vi "3458A Fetch from Digitizing Process.vi"(6 "stop ref":refnum<vi>, 7 "record start timestamp for time multiplex [s]":dbl, 8 "error in":errorcluster, 10 "Is last multiplexing cycle? (True)":bool=TRUE, 11 "session in":T3={"channels"=[], "sync unit"={"VISA"="", "type"=enum."Picotest U6200A"}, "awg unit"={"type"=enum."Agilent 331xxA to 332xxA", "VISA"="", "enable 10MHz ref"=FALSE, "cmi ckd2"={"VISA"="", "clock source"=enum."Auto", "manual ref clk"=FALSE, "ref clock [Hz]"=0.0, "div mode"=enum."Set divisor directly"}, "cmi sync v3"={"VISA"="", "baud rate [bd/s]"=115200, "source"=enum."Auto", "hv range"=enum."1kV", "fsrc is fixed"=FALSE, "fsrc [Hz]"=10000000.0, "freq integ [s]"=1.0, "freq filter"=5, "trig level"=enum."TTL 5V", "chn1 mode"=enum."Source divider", "chn1 level"=enum."Positive 5V", "chn2 mode"=enum."Source divider", "chn2 level"=enum."Positive 5V", "chn2 div"=1, "chn3 mode"=enum."Chn 1 Active", "chn3 level"=enum."Positive 5V", "chn1 div entry"=enum."Calculate nearest divisor from measured fx", "chn1 dev limit [%]"=1.0, "chn1 check dev"=FALSE}, "trigger"={"source"=enum."Immediate", "slope"=enum."POS", "coupling"=enum."DC", "level [V]"=0.0, "hysteresis [V]"=0.0, "pre-trigger [%]"=0.0}, "HMF2500 cfg"={"Baud Rate"=9600, "Parity"=0, "Data Bits"=8, "Flow Control"=4}}, "sync mode"=enum."MASTER-SLAVE, MASTER clocked by TIMER", "streaming mode"=FALSE, "idn mode"=enum."Auto", "sampling mode"=enum."DCV", "sample memory [B]"=0, "proc setup"={"channel id"=0, "packet size [smpl]"=0, "current timeout [s]"=0.0, "blk2blk timeout [s]"=0.0, "event time"=timestamp(0 s since 1904-01-01), "stop notifier"=refnum, "data queues"=[], "proc refs"=[], "bus semaphore"=refnum}, "sample size [B]"=0, "sample count"=0, "aux data"={"channel id"=0, "valid?"=[], "gain [V]"=[], "timestamp [s]"=[], "Ts [s]"=0.0, "abs timestamp"=timestamp(0 s since 1904-01-01), "t [deg C]"=[], "multiplex timestamp [s]"=-1.0, "only multiplex?"=FALSE, "multiplex smpl offset"=0, "overflow?"=FALSE}, "ranges [V]"=[], "aperture [s]"=0.0, "LEVEL trigger"={"edge"=enum."POS", "level [V]"=0.0, "coupling"=enum."DC"}, "trigger mode"=enum."AUTO", "measure temp.?"=FALSE, "disp mesages"=[], "shared bus?"=FALSE, "disable display?"=FALSE, "aper mode"=enum."Manual", "aper rules"=[], "multiplex"={"cycles"=0, "delay [s]"=0.0, "enabled"=FALSE, "overhead [s]"=1.0, "tot smpls"=0, "sub-rec"=0, "overhead [%]"=0.0, "emulated"=FALSE}, "F8588 lpf"=enum."Off", "F8588 pll"=enum."Off", "F8588 couple"=enum."DC, auto", "fs"={"freq mode"=enum."fs or Ts", "fs [Hz]"=0.0, "fref [Hz]"=0.0, "mul"=0.0, "div"=0.0}, "fs mode"=enum."fs or Ts"} {"awg unit"."HMF2500 cfg"."Flow Control" items=["None", "XON/XOFF", "RTS/CTS", "XON/XOFF & RTS/CTS", "DTR/DSR", "XON/XOFF & DTR/DSR"]; "awg unit"."HMF2500 cfg"."Data Bits" items=["7"=7, "8"=8]; "awg unit"."HMF2500 cfg"."Parity" items=["None", "Odd", "Even", "Mark", "Space"]; "awg unit"."HMF2500 cfg"."Baud Rate" items=["300"=300, "600"=600, "1200"=1200, "2400"=2400, "4800"=4800, "9600"=9600, "19200"=19200]; "awg unit"."cmi sync v3"."chn2 div" min=1 max=100000000 step=1; "awg unit"."cmi sync v3"."fsrc [Hz]" format="%_8p"; "channels"."Range [Vpk]" min=0.0}) -> (0 "error out":errorcluster, 1 "aux data":T1={"channel id"=0, "valid?"=[], "gain [V]"=[], "timestamp [s]"=[], "Ts [s]"=0.0, "abs timestamp"=timestamp(0 s since 1904-01-01), "t [deg C]"=[], "multiplex timestamp [s]"=-1.0, "only multiplex?"=FALSE, "multiplex smpl offset"=0, "overflow?"=FALSE}, 2 "data packet":T2, 3 "session out":T3={"channels"=[], "sync unit"={"VISA"="", "type"=enum."Picotest U6200A"}, "awg unit"={"type"=enum."Agilent 331xxA to 332xxA", "VISA"="", "enable 10MHz ref"=FALSE, "cmi ckd2"={"VISA"="", "clock source"=enum."Auto", "manual ref clk"=FALSE, "ref clock [Hz]"=0.0, "div mode"=enum."Set divisor directly"}, "cmi sync v3"={"VISA"="", "baud rate [bd/s]"=115200, "source"=enum."Auto", "hv range"=enum."1kV", "fsrc is fixed"=FALSE, "fsrc [Hz]"=10000000.0, "freq integ [s]"=1.0, "freq filter"=5, "trig level"=enum."TTL 5V", "chn1 mode"=enum."Source divider", "chn1 level"=enum."Positive 5V", "chn2 mode"=enum."Source divider", "chn2 level"=enum."Positive 5V", "chn2 div"=1, "chn3 mode"=enum."Chn 1 Active", "chn3 level"=enum."Positive 5V", "chn1 div entry"=enum."Calculate nearest divisor from measured fx", "chn1 dev limit [%]"=1.0, "chn1 check dev"=FALSE}, "trigger"={"source"=enum."Immediate", "slope"=enum."POS", "coupling"=enum."DC", "level [V]"=0.0, "hysteresis [V]"=0.0, "pre-trigger [%]"=0.0}, "HMF2500 cfg"={"Baud Rate"=9600, "Parity"=0, "Data Bits"=8, "Flow Control"=4}}, "sync mode"=enum."MASTER-SLAVE, MASTER clocked by TIMER", "streaming mode"=FALSE, "idn mode"=enum."Auto", "sampling mode"=enum."DCV", "sample memory [B]"=0, "proc setup"={"channel id"=0, "packet size [smpl]"=0, "current timeout [s]"=0.0, "blk2blk timeout [s]"=0.0, "event time"=timestamp(0 s since 1904-01-01), "stop notifier"=refnum, "data queues"=[], "proc refs"=[], "bus semaphore"=refnum}, "sample size [B]"=0, "sample count"=0, "aux data"={"channel id"=0, "valid?"=[], "gain [V]"=[], "timestamp [s]"=[], "Ts [s]"=0.0, "abs timestamp"=timestamp(0 s since 1904-01-01), "t [deg C]"=[], "multiplex timestamp [s]"=-1.0, "only multiplex?"=FALSE, "multiplex smpl offset"=0, "overflow?"=FALSE}, "ranges [V]"=[], "aperture [s]"=0.0, "LEVEL trigger"={"edge"=enum."POS", "level [V]"=0.0, "coupling"=enum."DC"}, "trigger mode"=enum."AUTO", "measure temp.?"=FALSE, "disp mesages"=[], "shared bus?"=FALSE, "disable display?"=FALSE, "aper mode"=enum."Manual", "aper rules"=[], "multiplex"={"cycles"=0, "delay [s]"=0.0, "enabled"=FALSE, "overhead [s]"=1.0, "tot smpls"=0, "sub-rec"=0, "overhead [%]"=0.0, "emulated"=FALSE}, "F8588 lpf"=enum."Off", "F8588 pll"=enum."Off", "F8588 couple"=enum."DC, auto", "fs"={"freq mode"=enum."fs or Ts", "fs [Hz]"=0.0, "fref [Hz]"=0.0, "mul"=0.0, "div"=0.0}, "fs mode"=enum."fs or Ts"} {"awg unit"."HMF2500 cfg"."Flow Control" items=["None", "XON/XOFF", "RTS/CTS", "XON/XOFF & RTS/CTS", "DTR/DSR", "XON/XOFF & DTR/DSR"]; "awg unit"."HMF2500 cfg"."Data Bits" items=["7"=7, "8"=8]; "awg unit"."HMF2500 cfg"."Parity" items=["None", "Odd", "Even", "Mark", "Space"]; "awg unit"."HMF2500 cfg"."Baud Rate" items=["300"=300, "600"=600, "1200"=1200, "2400"=2400, "4800"=4800, "9600"=9600, "19200"=19200]; "awg unit"."cmi sync v3"."chn2 div" min=1 max=100000000 step=1; "awg unit"."cmi sync v3"."fsrc [Hz]" format="%_8p"; "channels"."Range [Vpk]" min=0.0}, 4 "fetching done?":bool)   [LabVIEW 2020, in "3458A Virtual Digitizer.lvlib"]
doc: "This VI fetches digitized samples from the digitizing processes initiated by 'Initiate Digitizing Process'. It checks the data queues of the particular channels and merges samples from the channels into 2D array whenever all channels return matching series of samples. Until all channels sends some samples to the queues it won't return data but also won't return error. When some of the digitizing processes exits with error or exits prematurely it will generate error. It will also generate error when fetching timeout occures. When processes seems to returnes unsynchronized data it will also generate error and terminate fetching. Called of this vi must keep checking flag 'valid?' in the 'data packet' and 'aux data'. When the flag is True the data must be checked/collected. When this VI returnes 'fetching done?' or error flag the caller shall not call the function again.\n\nFor multiplexing mode and not 'Is last multiplex cycle?' it will only wait to emulate recording and returns 'Fetching done'. It will only fetch in the last multiplex cycle (default)."
uses:
  3458A Virtual Digitizer.lvlib
  3458A Digitizer Session.ctl
  3458A Virtual Channel Config.ctl
  Counter/Counter Session.ctl
  Counter/Counter Type.ctl
  AWG/AWG Session.ctl
  AWG/AWG Type.ctl
  AWG/CMI Clock Divider v2/CMI ckd2 Session.ctl
  AWG/CMI Clock Divider v2/CMI ckd2 Source Mode.ctl
  AWG/CMI Clock Divider v2/CMI ckd2 Divisor Mode.ctl
  AWG/CMI Sync V3/CMI Sync V3 session.ctl
  AWG/CMI Sync V3/Configure/CMI Sync V3 Reference Clock Source.ctl
  AWG/CMI Sync V3/Configure/CMI Sync V3 HV input Range.ctl
  AWG/CMI Sync V3/Configure/CMI Sync V3 Trigger Input Level.ctl
  AWG/CMI Sync V3/Configure/CMI Sync V3 Channel 1 Mode.ctl
  AWG/CMI Sync V3/Configure/CMI Sync V3 Channel Output Levels.ctl
  AWG/CMI Sync V3/Configure/CMI Sync V3 Channel 2 Mode.ctl
  AWG/CMI Sync V3/Configure/CMI Sync V3 Channel 3 Mode.ctl
  AWG/CMI Sync V3/Configure/CMI Sync V3 Channel 1 Divisor Entry Mode.ctl
  adc/ADC Trig Config.ctl
  adc/ADC Trig Mode Source.ctl
  adc/ADC Trig Slope.ctl
  adc/ADC Trig Coupling.ctl
  AWG/RaS HMF2500/HMF2500 Config.ctl
  3458A Sync Mode.ctl
  3458A Idn Mode.ctl
  3458A Digitizing Low Levels/Configure/Sampling Mode.ctl
  3458A Digitizing Process Options.ctl
  3458A Data Packet.ctl
  3458A Aux Record Data.ctl
  3458A Digitizing Low Levels/Configure/Level Setup.ctl
  3458A Digitizing Low Levels/Configure/First Sample Trigger.ctl
  3458A Aperture Selection Mode.ctl
  3458A Multiplexing Config.ctl
  Fluke 8588A/F8588A Low Pass Filter.ctl
  Fluke 8588A/F8588A Phase Lock.ctl
  Fluke 8588A/F8588A Coupling.ctl
  3458A Sampling Rate.ctl
  AWG/AWG Clock Setup Mode.ctl
  3458A Sample Rate Mode.ctl
  <vilib>/Utility/error.llb/Error Cluster From Error Code.vi
  <vilib>/ErrorRing/Error Ring.xnode
  varilib/varilib.lvlib
  AWG/AWG.lvlib
  Counter/Counter.lvlib
  3458A Digitizing Low Levels/3458A Digitizing Low Levels.lvlib
  AWG/CMI Sync V3/CMI Sync Unit V3.lvlib
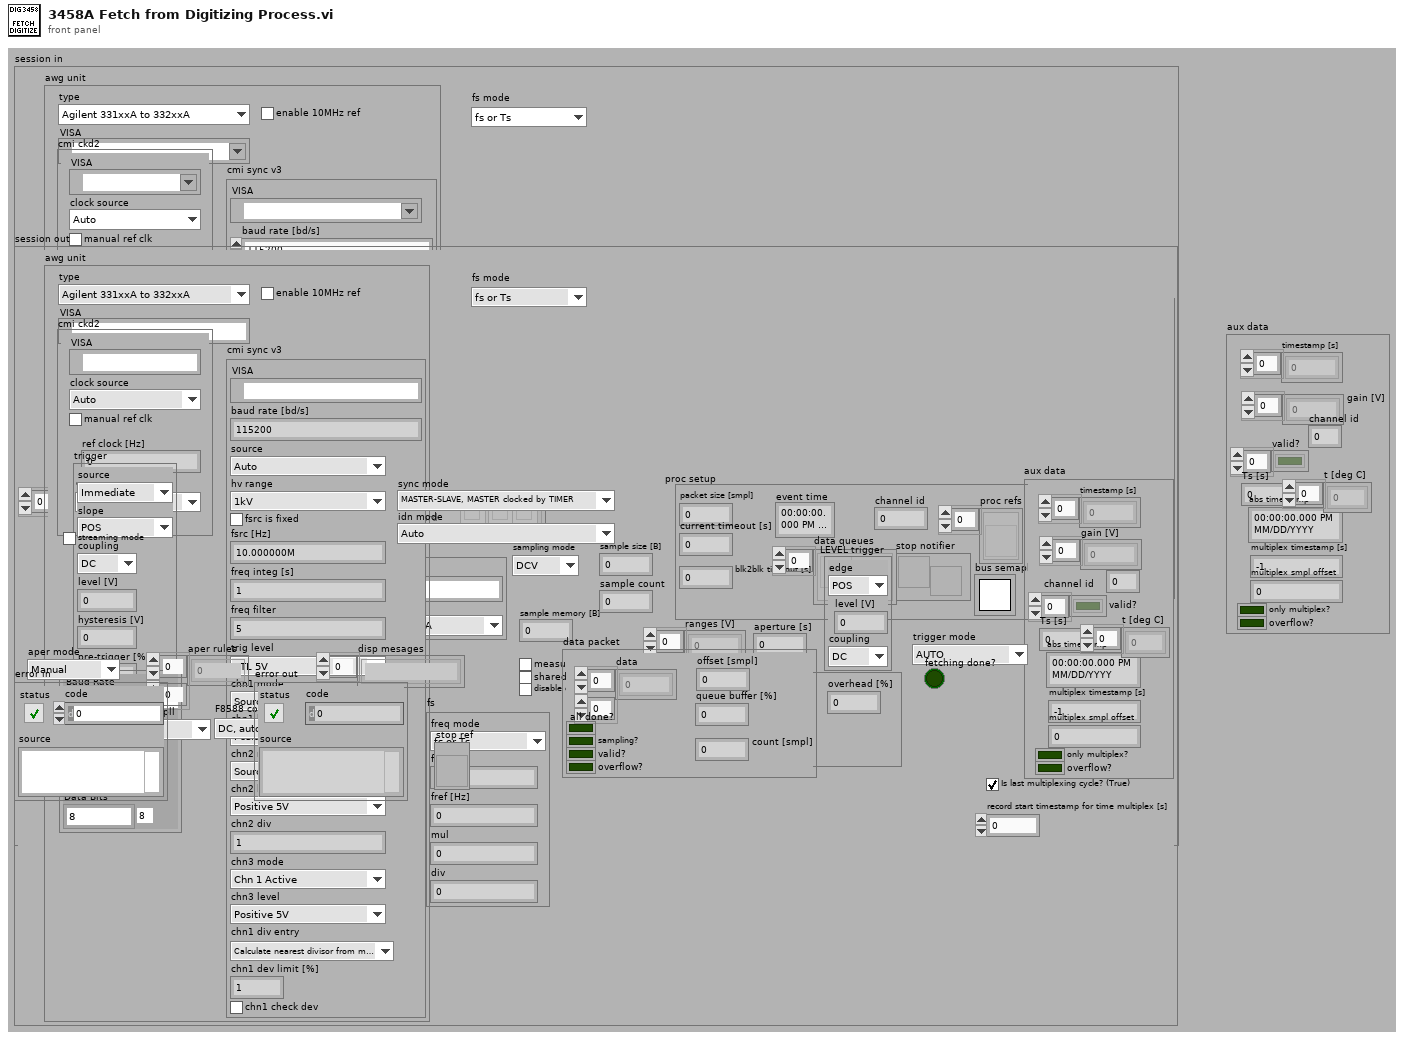
[diagram p1: front panel]
types:
  T1 = typedef "3458A Virtual Digitizer.lvlib/3458A Aux Record Data.ctl" = cluster{"channel id":i32, "valid?":bool[], "gain [V]":dbl[], "timestamp [s]":dbl[], "Ts [s]":dbl, "abs timestamp":timestamp, "t [deg C]":dbl[], "multiplex timestamp [s]":dbl, "only multiplex?":bool, "multiplex smpl offset":i64, "overflow?":bool}
  T2 = typedef "3458A Virtual Digitizer.lvlib/3458A Data Packet.ctl" = cluster{"data":i32[][], "offset [smpl]":i32, "count [smpl]":i32, "all done?":bool, "sampling?":bool, "queue buffer [%]":dbl, "valid?":bool, "overflow?":bool}
  T3 = typedef "3458A Virtual Digitizer.lvlib/3458A Digitizer Session.ctl" = cluster{"channels":T4[], "sync unit":T5, "awg unit":T7, "sync mode":T26, "streaming mode":bool, "idn mode":T27, "sampling mode":T28, "sample memory [B]":i32, "proc setup":T29, "sample size [B]":i32, "sample count":i32, "aux data":T1, "ranges [V]":dbl[], "aperture [s]":dbl, "LEVEL trigger":T31, "trigger mode":T32, "measure temp.?":bool, "disp mesages":string[], "shared bus?":bool, "disable display?":bool, "aper mode":T33, "aper rules":dbl[][], "multiplex":T34, "F8588 lpf":T35, "F8588 pll":T36, "F8588 couple":T37, "fs":T38, "fs mode":T40}
  T4 = typedef "3458A Virtual Digitizer.lvlib/3458A Virtual Channel Config.ctl" = cluster{"VISA":refnum<visa-resource-name>, "Range [Vpk]":dbl, "btn clr":bool, "btn up":bool, "btn down":bool, "F8588":bool, "F8588 guard":bool}
  T5 = typedef "Counter.lvlib/Counter Session.ctl" = cluster{"VISA":refnum<visa-resource-name>, "type":T6}
  T6 = typedef "Counter.lvlib/Counter Type.ctl" = enum16{"Picotest U6200A", "dummy"}
  T7 = typedef "AWG.lvlib/AWG Session.ctl" = cluster{"type":T8, "VISA":refnum<visa-resource-name>, "enable 10MHz ref":bool, "cmi ckd2":T9, "cmi sync v3":T12, "trigger":T21, "HMF2500 cfg":T25}
  T8 = typedef "AWG.lvlib/AWG Type.ctl" = enum16{"Agilent 331xxA to 332xxA", "Agilent 335xxA to 336xxA", "Tektronix AFG3101C", "R&S HMF25xx", "CMI Clock Divider v2", "CMI Sync Unit V3", "dummy"}
  T9 = typedef "AWG.lvlib/CMI ckd2 Session.ctl" = cluster{"VISA":refnum<visa-resource-name>, "clock source":T10, "manual ref clk":bool, "ref clock [Hz]":dbl, "div mode":T11}
  T10 = typedef "AWG.lvlib/CMI ckd2 Source Mode.ctl" = enum16{"Auto", "LF clock", "HF clock", "Internal"}
  T11 = typedef "AWG.lvlib/CMI ckd2 Divisor Mode.ctl" = enum16{"Set divisor directly", "Set divisor by frequency"}
  T12 = typedef "AWG.lvlib/CMI Sync Unit V3.lvlib/CMI Sync V3 session.ctl" = cluster{"VISA":refnum<visa-resource-name>, "baud rate [bd/s]":i32, "source":T13, "hv range":T14, "fsrc is fixed":bool, "fsrc [Hz]":dbl, "freq integ [s]":dbl, "freq filter":i32, "trig level":T15, "chn1 mode":T16, "chn1 level":T17, "chn2 mode":T18, "chn2 level":T17, "chn2 div":i32, "chn3 mode":T19, "chn3 level":T17, "chn1 div entry":T20, "chn1 dev limit [%]":dbl, "chn1 check dev":bool}
  T13 = typedef "AWG.lvlib/CMI Sync Unit V3.lvlib/CMI Sync V3 Reference Clock Source.ctl" = enum16{"Auto", "Internal", "Logic", "Sine", "HV"}
  T14 = typedef "AWG.lvlib/CMI Sync Unit V3.lvlib/CMI Sync V3 HV input Range.ctl" = enum16{"10V", "60V", "250V", "1kV"}
  T15 = typedef "AWG.lvlib/CMI Sync Unit V3.lvlib/CMI Sync V3 Trigger Input Level.ctl" = enum16{"LVCMOS 3V3", "TTL 5V"}
  T16 = typedef "AWG.lvlib/CMI Sync Unit V3.lvlib/CMI Sync V3 Channel 1 Mode.ctl" = enum16{"Source divider", "DDS absolute", "DDS ratio", "DDS ratio M/N"}
  T17 = typedef "AWG.lvlib/CMI Sync Unit V3.lvlib/CMI Sync V3 Channel Output Levels.ctl" = enum16{"Positive 3V3", "Negative 3V3", "Positive 5V", "Negative 5V"}
  T18 = typedef "AWG.lvlib/CMI Sync Unit V3.lvlib/CMI Sync V3 Channel 2 Mode.ctl" = enum16{"Source divider", "Chn 1 divide"}
  T19 = typedef "AWG.lvlib/CMI Sync Unit V3.lvlib/CMI Sync V3 Channel 3 Mode.ctl" = enum16{"Chn 1 Active", "Chn 2 Active", "Chn 1 Trigger", "Chn 2 Trigger", "Gate", "PPS", "10MHz"}
  T20 = typedef "AWG.lvlib/CMI Sync Unit V3.lvlib/CMI Sync V3 Channel 1 Divisor Entry Mode.ctl" = enum16{"Set divisor directly", "Calculate nearest divisor from measured fx"}
  T21 = typedef "ADC Trig Config.ctl" = cluster{"source":T22, "slope":T23, "coupling":T24, "level [V]":dbl, "hysteresis [V]":dbl, "pre-trigger [%]":dbl}
  T22 = typedef "ADC Trig Mode Source.ctl" = enum16{"Immediate", "External", "Level"}
  T23 = typedef "ADC Trig Slope.ctl" = enum16{"POS", "NEG"}
  T24 = typedef "ADC Trig Coupling.ctl" = enum16{"DC", "AC"}
  T25 = typedef "AWG.lvlib/HMF2500 Config.ctl" = cluster{"Baud Rate":u32, "Parity":u16, "Data Bits":u16, "Flow Control":u16}
  T26 = typedef "3458A Virtual Digitizer.lvlib/3458A Sync Mode.ctl" = enum16{"MASTER-SLAVE, MASTER clocked by TIMER", "MASTER-SLAVE, MASTER clocked by AWG", "ALL clocked by AWG", "MASTER-SLAVE, ALL clocked by TIMER", "ALL clocked by AWG with DFLL"}
  T27 = typedef "3458A Virtual Digitizer.lvlib/3458A Idn Mode.ctl" = enum16{"Auto", "Sequential (chn A, chn B, ...)", "From calibration string"}
  T28 = typedef "3458A Virtual Digitizer.lvlib/3458A Digitizing Low Levels.lvlib/Sampling Mode.ctl" = enum16{"DCV", "DSDC", "DSAC"}
  T29 = typedef "3458A Virtual Digitizer.lvlib/3458A Digitizing Process Options.ctl" = cluster{"channel id":i32, "packet size [smpl]":i32, "current timeout [s]":dbl, "blk2blk timeout [s]":dbl, "event time":timestamp, "stop notifier":refnum<notifier>, "data queues":refnum<queue>[], "proc refs":refnum<vi>[], "bus semaphore":T30}
  T30 = typedef "Semaphore RefNum" = refnum<k1>
  T31 = typedef "3458A Virtual Digitizer.lvlib/3458A Digitizing Low Levels.lvlib/Level Setup.ctl" = cluster{"edge":enum16{"POS", "NEG"}, "level [V]":dbl, "coupling":enum16{"DC", "AC"}}
  T32 = typedef "3458A Virtual Digitizer.lvlib/3458A Digitizing Low Levels.lvlib/First Sample Trigger.ctl" = enum16{"AUTO", "EXT", "SYN", "SGL", "HOLD", "LEVEL"}
  T33 = typedef "3458A Virtual Digitizer.lvlib/3458A Aperture Selection Mode.ctl" = enum16{"Manual", "Maximum", "Table"}
  T34 = typedef "3458A Virtual Digitizer.lvlib/3458A Multiplexing Config.ctl" = cluster{"cycles":i32, "delay [s]":dbl, "enabled":bool, "overhead [s]":dbl, "tot smpls":i64, "sub-rec":i32, "overhead [%]":dbl, "emulated":bool}
  T35 = typedef "F8588A Low Pass Filter.ctl" = enum16{"Off", "100 kHz", "3 MHz"}
  T36 = typedef "F8588A Phase Lock.ctl" = enum16{"Off", "1 MHz", "10 MHz"}
  T37 = typedef "F8588A Coupling.ctl" = enum16{"AC, 1 MOhm", "AC, 10 MOhm", "DC, 1 MOhm", "DC, 10 MOhm", "DC, auto"}
  T38 = typedef "3458A Virtual Digitizer.lvlib/3458A Sampling Rate.ctl" = cluster{"freq mode":T39, "fs [Hz]":dbl, "fref [Hz]":dbl, "mul":dbl, "div":dbl}
  T39 = typedef "AWG.lvlib/AWG Clock Setup Mode.ctl" = enum16{"fs or Ts", "fs or Ts with fref", "fref/N", "fref*M/N", "fref*Ratio"}
  T40 = typedef "3458A Sample Rate Mode.ctl" = enum16{"fs or Ts", "fs*M/N"}
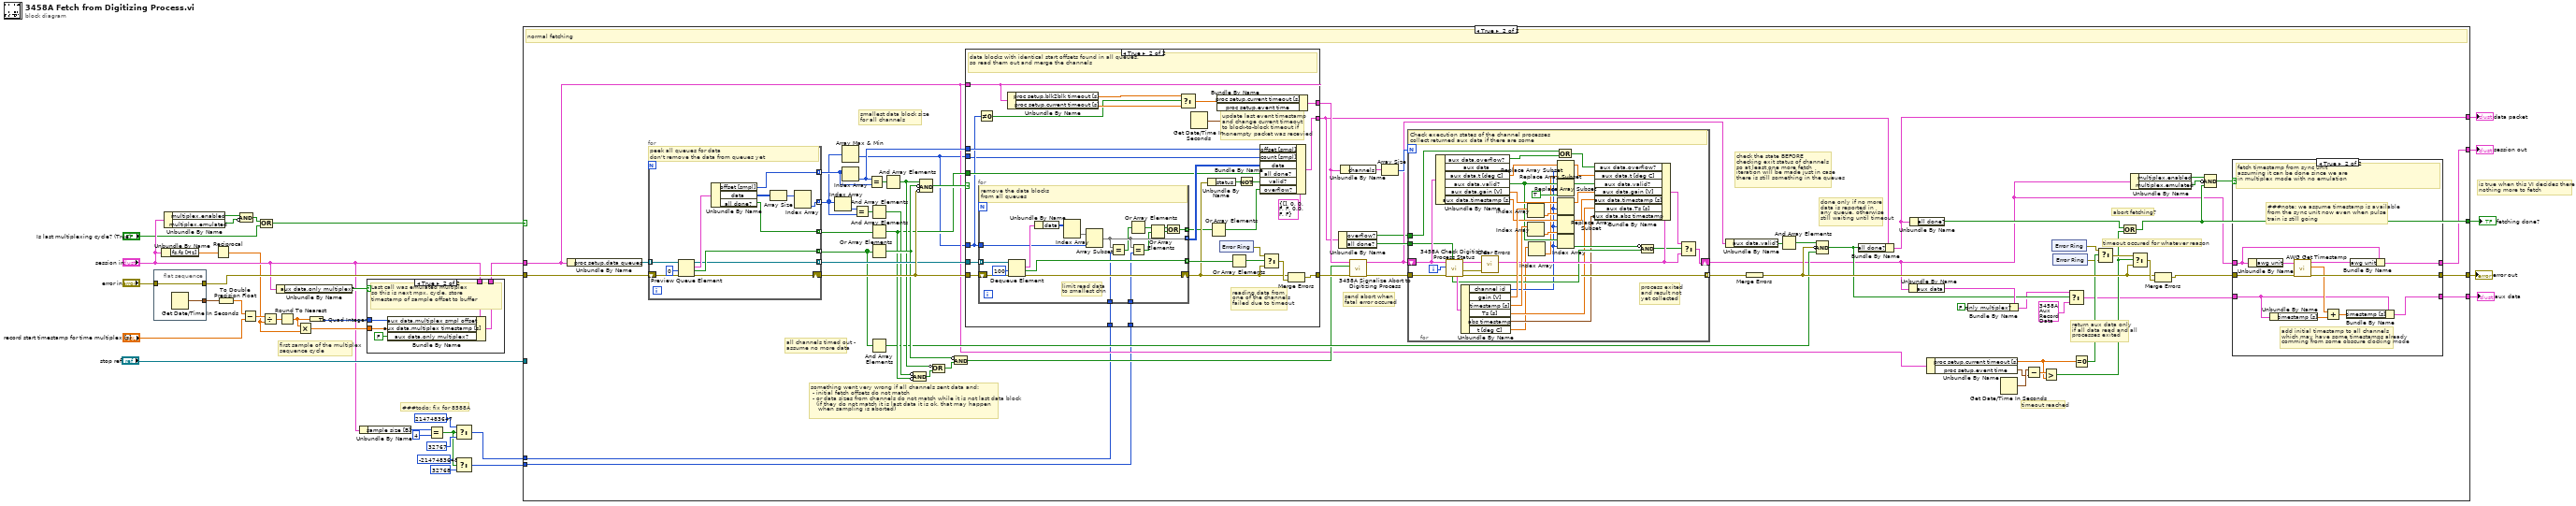
[diagram p0: block diagram]
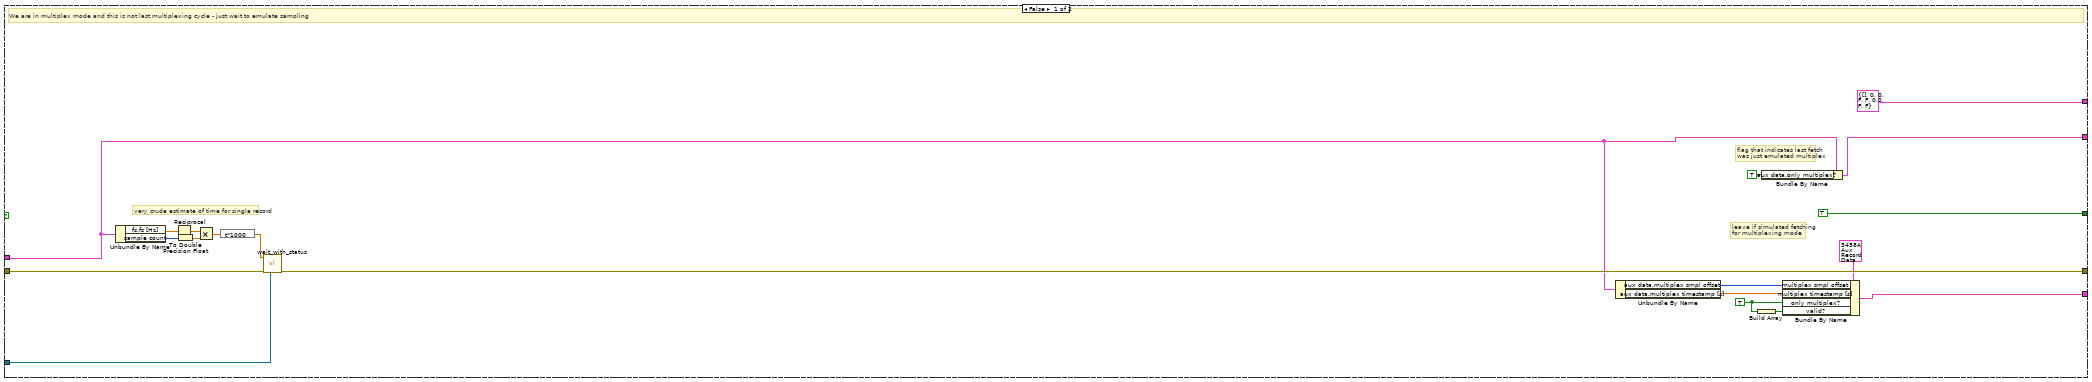
[diagram p3: hidden frame]
diagram:
  # "###todo: fix for 8588A"
  # "first sample of the multiplex\nsequence cycle"
  # "is true when this VI decides there is\nnothing more to fetch"
  n1 = flat-sequence {
    tunnel: [w37] -> w23
    tunnel: "error in" -> [w37]
    tunnel: [w36] -> w26
    frame #0 {
      n2 = Get Date/Time In Seconds() -> (seconds since 1Jan1904=w36:timestamp)
    }
  }
  n3 = Unbundle By Name("session in") -> ("fs.fs [Hz]"=w21:dbl)
  n4 = Unbundle By Name("session in") -> ("multiplex.enabled"=w6:bool, "multiplex.emulated"=w5:bool)
  n5 = Reciprocal(x=w21) -> (1/x=w1:dbl)
  n6 = To Double Precision Float(number=w26) -> (double precision float=w27:dbl)
  n7 = Compound Arithmetic op=AND(w6, invert w5) -> (w4:bool)
  n8 = Subtract(x=w27, y="record start timestamp for time multiplex [s]") -> (x-y=w28:dbl)
  n9 = Compound Arithmetic op=OR(w4, "Is last multiplexing cycle? (True)") -> (w2:bool)
  n10 = Divide(x=w28, y=w1) -> (x/y=w29:dbl)
  n11 = Unbundle By Name("session in") -> ("aux data.only multiplex?"=w19:bool)
  n12 = Round To Nearest(number=w29) -> (nearest integer value=w22:dbl)
  n13 = Multiply(x=w22, y=w1) -> (x*y=w17:dbl)
  n14 = To Quad Integer(1:w22) -> (0:w18:i64)
  n15 = Unbundle By Name("session in") -> ("sample size [B]"=w16:i32)
  n16 = case shown="True" w19 {
    tunnel: "session in" -> [w38 w43]
    tunnel: [w38 w42] -> w20
    tunnel: w18 -> [_ w40]
    tunnel: w17 -> [_ w39]
    frame False {
      # "regular fetch - do nothing"
    }
    frame True {
      # "Last call was emulated multiplex\nso this is next mpx. cycle, store\ntimestamp of sample offset to buffer"
      n17 = Bundle By Name(cluster=w43, "aux data.multiplex smpl offset"=w40, "aux data.multiplex timestamp [s]"=w39, "aux data.only multiplex?"=FALSE) -> (w42:T3)
    }
  }
  n18 = Equal?(x=w16, y=4) -> (x = y?=w12:bool)
  n19 = Select(t=2147483647 ("y"), s=w12, f=32767 ("y")) -> (s? t:f=w8:i32)
  n20 = Select(t=-2147483648 ("y"), s=w12, f=32768 ("y")) -> (s? t:f=w9:i32)
  n21 = case shown="True" w2 {
    tunnel: w23 -> [w56 w128]
    tunnel: [w60 w70] -> w35
    tunnel: w20 -> [w49 w81]
    tunnel: [w51 w66] -> w34
    tunnel: "stop ref" -> [w59 _]
    tunnel: [TRUE w68] -> w32
    tunnel: [w54 w64] -> w31
    tunnel: [T2 {"data"=[], "offset [smpl]"=0, "count [smpl]"=0, "all done?"=FALSE, "sampling?"=FALSE, "queue buffer [%]"=0.0, "valid?"=FALSE, "overflow?"=FALSE} ("niScope packet") w79] -> w30
    tunnel: w9 -> [_ w75]
    tunnel: w8 -> [_ w76]
    frame False {
      w52 = TRUE ("only multiplex?")
      # "flag that indicates last fetch\nwas just emulated multiplex"
      # "leave if simulated fetching\nfor multiplexing mode"
      # "very crude estimate of time for single record"
      # "We are in multiplex mode and this is not last multiplexing cycle - just wait to emulate sampling"
      n22 = Unbundle By Name(w49) -> ("fs.fs [Hz]"=w57:dbl, "sample count"=w63:i32)
      n23 = Reciprocal(x=w57) -> (1/x=w44:dbl)
      n24 = To Double Precision Float(number=w63) -> (double precision float=w62:dbl)
      n25 = Multiply(x=w44, y=w62) -> (x*y=w61:dbl)
      n26 = expression code="t*1000"(w61) -> (w45:dbl)
      n27 = call "wait_with_status.vi"("stop ref"=w59, "error in"=w56, "ms to wait"=w45) -> ("error out"=w60:errorcluster)  [unwired: 8 in]
      n28 = Unbundle By Name(w49) -> ("aux data.multiplex smpl offset"=w48:i64, "aux data.multiplex timestamp [s]"=w47:dbl)
      n29 = Build Array(w52) -> (w53:bool[])
      n30 = Bundle By Name(cluster=w49, "aux data.only multiplex?"=TRUE) -> (w51:T3)
      n31 = Bundle By Name(cluster=T1 {"channel id"=0, "valid?"=[], "gain [V]"=[], "timestamp [s]"=[], "Ts [s]"=0.0, "abs timestamp"=timestamp(0 s since 1904-01-01), "t [deg C]"=[], "multiplex timestamp [s]"=0.0, "only multiplex?"=FALSE, "multiplex smpl offset"=0, "overflow?"=FALSE} ("f"), "multiplex smpl offset"=w48, "multiplex timestamp [s]"=w47, "only multiplex?"=w52, "valid?"=w53) -> (w54:T1)
    }
    frame True {
      # "abort fetching?"
      # "check the state BEFORE\nchecking exit status of channels \nso at least one more fetch\niteration will be made just in case \nthere is still something in the queues"
      # "return aux data only\nif all data read and all\nprocesses exited"
      # "done only if no more\ndata is reported in\nany queue, otherwise\nstill waiting until timeout"
      # "timeout reached"
      # "send abort when\nfatal error occured"
      # "something went very wrong if all channels sent data and:\n - initial fetch offsets do not match\n - or data sizes from channels do not match while it is not last data block\n   (if they do not match it is last data it is ok, that may happen\n    when sampling is aborted)"
      # "all channels timed out -\nassume no more data"
      # "timeout occured for whatever reason"
      # "smallest data block size\nfor all channels"
      # "normal fetching"
      n32 = Unbundle By Name(w81) -> ("proc setup.data queues"=w101:refnum<queue>[])
      n33 = for {
        tunnel: w101 -> [w249] mode=indexing
        tunnel: [w246] -> w113 mode=indexing
        tunnel: [w239] -> w123 mode=indexing
        tunnel: [w242] -> w127 mode=indexing
        shift-right: [w247] -> w121
        shift-left: w128 -> [w250]
        tunnel: [w241] -> w122 mode=indexing
        tunnel: [w240] -> w120 mode=indexing
        # "peek all queues for data\ndon't remove the data from queues yet"
        n34 = Preview Queue Element(queue=w249, timeout in ms (-1)=0, error in (no error)=w250) -> (queue out=w240:refnum<queue>, element=w245:T2, timed out?=w246:bool, error out=w247:errorcluster)
        n35 = Unbundle By Name(w245) -> ("offset [smpl]"=w242:i32, "data"=w244:i32[][], "all done?"=w241:bool)
        n36 = Array Size(array=w244) -> (size(s)=w243:i32[])
        n37 = Index Array(array=w243) -> (element #2=w239:i32)  [unwired: 2 in, 1 out]
      }
      n38 = Index Array(array=w123) -> (element=w124:i32)  [unwired: 1 in]
      n39 = Array Max & Min(array=w123) -> (min value=w80:i32)  [unwired: 3 out]
      n40 = Index Array(array=w127) -> (element=w118:i32)  [unwired: 1 in]
      n41 = Equal?(x=w124, y=w123) -> (x = y?=w125:bool[])
      n42 = Equal?(x=w118, y=w127) -> (x = y?=w126:bool[])
      n43 = And Array Elements(Boolean array=w125) -> (logical AND=w108:bool)
      n44 = And Array Elements(Boolean array=w122) -> (logical AND=w107:bool)
      n45 = Or Array Elements(Boolean array=w113) -> (logical OR=w112:bool)
      n46 = And Array Elements(Boolean array=w113) -> (logical AND=w96:bool)
      n47 = And Array Elements(Boolean array=w126) -> (logical AND=w110:bool)
      n48 = Compound Arithmetic op=AND(invert w108, invert w107) -> (w109:bool)
      n49 = Compound Arithmetic op=AND(w110, invert w112, invert w121) -> (w119:bool)
      n50 = Compound Arithmetic op=OR(invert w110, w109) -> (w111:bool)
      n51 = Compound Arithmetic op=AND(invert w112, w111) -> (w82:bool)
      n52 = case shown="True" w119 {
        tunnel: w121 -> [w188 w216]
        tunnel: w120 -> [_ w215]
        tunnel: [w188 w210] -> w106
        tunnel: w80 -> [_ w203]
        tunnel: w107 -> [_ w207]
        tunnel: w118 -> [_ w206]
        tunnel: [_ w205] -> w94
        tunnel: w81 -> [w187 w201]
        tunnel: [w187 w204] -> w104
        tunnel: w80 -> [_ w193]
        tunnel: w76 -> [_ w192]
        tunnel: w75 -> [_ w191]
        frame False {
          # "error or read data offsets of from various channels do not match"
        }
        frame True {
          # "update last event timestamp\nand change current timeout\nto block-to-block timeout if\nnonempty packet was recevied"
          # "reading data from\none of the channels\nfailed due to timeout"
          # "data blocks with identical start offsets found in all queues,\nso read them out and merge the channels"
          n53 = Not Equal To 0?(x=w203) -> (x != 0?=w198:bool)
          n54 = for {
            tunnel: w215 -> [w237] mode=indexing
            tunnel: [w234] -> w214 mode=indexing
            shift-right: [w235] -> w196
            shift-left: w216 -> [w238]
            tunnel: w203 -> [w232]
            tunnel: [w228] -> w208 mode=indexing
            tunnel: w192 -> [w229]
            tunnel: w191 -> [w227]
            tunnel: [w222] -> w190 mode=indexing
            # "limit read data\nto smallest chn"
            # "remove the data blocks\nfrom all queues"
            n55 = Dequeue Element(queue=w237, timeout in ms (-1)=100, error in (no error)=w238) -> (element=w233:T2, timed out?=w234:bool, error out=w235:errorcluster)  [unwired: 1 out]
            n56 = Unbundle By Name(w233) -> ("data"=w231:i32[][])
            n57 = Index Array(array=w231) -> (element=w230:i32[])  [unwired: 2 in]
            n58 = Array Subset(array=w230, length=w232) -> (w228:i32[])  [unwired: 1 in]
            n59 = Equal?(x=w228, y=w229) -> (x = y?=w225:bool[])
            n60 = Or Array Elements(Boolean array=w225) -> (logical OR=w223:bool)
            n61 = Equal?(x=w228, y=w227) -> (x = y?=w226:bool[])
            n62 = Or Array Elements(Boolean array=w226) -> (logical OR=w224:bool)
            n63 = Compound Arithmetic op=OR(w223, w224) -> (w222:bool)
          }
          n64 = Unbundle By Name(w201) -> ("proc setup.blk2blk timeout [s]"=w200:dbl, "proc setup.current timeout [s]"=w199:dbl)
          n65 = Select(t=w200, s=w198, f=w199) -> (s? t:f=w197:dbl)
          n66 = Get Date/Time In Seconds() -> (seconds since 1Jan1904=w202:timestamp)
          n67 = Unbundle By Name(w196) -> ("status"=w195:bool)
          n68 = Or Array Elements(Boolean array=w190) -> (logical OR=w189:bool)
          n69 = Bundle By Name(cluster=w201, "proc setup.current timeout [s]"=w197, "proc setup.event time"=w202) -> (w204:T3)
          n70 = xnode "Error Ring"() -> ("error out"=w212:errorcluster)
          n71 = Or Array Elements(Boolean array=w214) -> (logical OR=w213:bool)
          n72 = Not(x=w195) -> (.not. x?=w194:bool)
          n73 = Bundle By Name(cluster=T2 {"data"=[], "offset [smpl]"=0, "count [smpl]"=0, "all done?"=FALSE, "sampling?"=FALSE, "queue buffer [%]"=0.0, "valid?"=FALSE, "overflow?"=FALSE} ("niScope packet"), "offset [smpl]"=w206, "count [smpl]"=w193, "data"=w208, "all done?"=w207, "valid?"=w194, "overflow?"=w189) -> (w205:T2)
          n74 = Select(t=w212, s=w213, f=w196) -> (s? t:f=w211:errorcluster)
          n75 = Merge Errors(w196, w211) -> (w210:errorcluster)
        }
      }
      n76 = Unbundle By Name(w94) -> ("overflow?"=w74:bool, "all done?"=w93:bool)
      n77 = Unbundle By Name(w104) -> ("channels"=w117:T4[])
      n78 = call "3458A Signalize Abort to Digitizing Process.vi"("error in"=w106, "send abort signal? (True)"=w82, "session in"=w104) -> ("error out (copy)"=w105:errorcluster, "session out"=w90:T3)  [unwired: 7 in]
      n79 = Array Size(array=w117) -> (size(s)=w114:i32)
      n80 = for {
        N: w114 -> [_]
        tunnel: w105 -> [w186]
        tunnel: [w164] -> w116 mode=indexing
        shift-right: [w166] -> w67
        shift-left: w90 -> [w176]
        tunnel: w93 -> [w165]
        tunnel: w74 -> [w153]
        i -> [w185]
        # "process exited\nand result not \nyet collected"
        # "Check execution states of the channel processes\ncollect returned aux data if there are some"
        n81 = Unbundle By Name(w176) -> ("aux data.overflow?"=w155:bool, "aux data.t [deg C]"=w158:dbl[], "aux data.valid?"=w170:bool[], "aux data.gain [V]"=w182:dbl[], "aux data.timestamp [s]"=w177:dbl[])  [unwired: 1 out]
        n82 = call "3458A Check Digitizing Process Status.vi"("wait for exit (False)"=w165, "error in"=w186, "channel id"=w185, "digitizer session in"=w176) -> ("error out"=w164:errorcluster, "proc error out"=w163:errorcluster, "digitizer session out"=w172:T3, "aux data out"=w184:T1, "aux data valid?"=w169:bool)  [unwired: 2 in, 1 out]
        n83 = Unbundle By Name(w184) -> ("channel id"=w159:i32, "gain [V]"=w181:dbl[], "timestamp [s]"=w179:dbl[], "Ts [s]"=w162:dbl, "abs timestamp"=w161:timestamp, "t [deg C]"=w157:dbl[])
        n84 = call <vilib>:"Clear Errors.vi"("error in (no error)"=w163) -> ()  [unwired: 5 in, 2 out]
        n85 = Index Array(array=w181) -> (element=w180:dbl)  [unwired: 1 in]
        n86 = Index Array(array=w179) -> (element=w178:dbl)  [unwired: 1 in]
        n87 = Index Array(array=w157) -> (element=w156:dbl)  [unwired: 1 in]
        n88 = Replace Array Subset(array=w158, new element=w156, index=w159) -> (w160:dbl[])
        n89 = Replace Array Subset(array=w170, new element=TRUE ("new element/subarray"), index=w159) -> (w175:bool[])
        n90 = Replace Array Subset(array=w182, new element=w180, index=w159) -> (w174:dbl[])
        n91 = Replace Array Subset(array=w177, new element=w178, index=w159) -> (w171:dbl[])
        n92 = Index Array(array=w170, index=w159) -> (element=w168:bool)
        n93 = Compound Arithmetic op=OR(w153, w155) -> (w154:bool)
        n94 = Bundle By Name(cluster=w172, "aux data.overflow?"=w154, "aux data.t [deg C]"=w160, "aux data.valid?"=w175, "aux data.gain [V]"=w174, "aux data.timestamp [s]"=w171, "aux data.Ts [s]"=w162, "aux data.abs timestamp"=w161) -> (w173:T3)
        n95 = Compound Arithmetic op=AND(invert w168, w169) -> (w167:bool)
        n96 = Select(t=w173, s=w167, f=w172) -> (s? t:f=w166:T3)
      }
      n97 = Unbundle By Name(w90) -> ("aux data.valid?"=w100:bool[])
      n98 = Merge Errors(w116) -> (w102:errorcluster)
      n99 = And Array Elements(Boolean array=w100) -> (logical AND=w99:bool)
      n100 = Compound Arithmetic op=AND(w99, invert w102, w96) -> (w95:bool)
      n101 = Bundle By Name(cluster=w94, "all done?"=w95) -> (w79:T2)
      n102 = Unbundle By Name(w67) -> ("aux data"=w98:T1)
      n103 = Unbundle By Name(w79) -> ("all done?"=w83:bool)
      n104 = Unbundle By Name(w81) -> ("proc setup.current timeout [s]"=w88:dbl, "proc setup.event time"=w91:timestamp)
      n105 = Bundle By Name(cluster=w98, "only multiplex?"=FALSE) -> (w78:T1)
      n106 = Get Date/Time In Seconds() -> (seconds since 1Jan1904=w92:timestamp)
      n107 = Subtract(x=w92, y=w91) -> (x-y=w103:dbl)
      n108 = Greater?(x=w103, y=w88) -> (0:w84:bool)
      n109 = xnode "Error Ring"() -> ("error out"=w85:errorcluster)
      n110 = xnode "Error Ring"() -> ("error out"=w86:errorcluster)
      n111 = Select(t=w78, s=w95, f=T1 {"channel id"=0, "valid?"=[], "gain [V]"=[], "timestamp [s]"=[], "Ts [s]"=0.0, "abs timestamp"=timestamp(0 s since 1904-01-01), "t [deg C]"=[], "multiplex timestamp [s]"=-1.0, "only multiplex?"=FALSE, "multiplex smpl offset"=0, "overflow?"=FALSE}) -> (s? t:f=w65:T1)
      n112 = Equal To 0?(x=w88) -> (x = 0?=w87:bool)
      n113 = Select(t=w85, s=w87, f=w86) -> (s? t:f=w89:errorcluster)
      n114 = Compound Arithmetic op=OR(w83, w84) -> (w68:bool)
      n115 = Unbundle By Name(w67) -> ("multiplex.enabled"=w73:bool, "multiplex.emulated"=w72:bool)
      n116 = Select(t=w89, s=w84, f=w102) -> (s? t:f=w115:errorcluster)
      n117 = Merge Errors(w102, w115) -> (w71:errorcluster)
      n118 = Compound Arithmetic op=AND(w73, invert w72, w68) -> (w69:bool)
      n119 = case shown="True" w69 {
        tunnel: w71 -> [w131 w142]
        tunnel: [w131 w141] -> w70
        tunnel: w67 -> [w130 w139]
        tunnel: [w130 w137] -> w66
        tunnel: w65 -> [w129 w134]
        tunnel: [w129 w132] -> w64
        frame False {
        }
        frame True {
          # "###note: we assume timestamp is available\nfrom the sync unit now even when pulse\ntrain is still going"
          # "add initial timestamp to all channels\nwhich may have some timestamps already\ncomming from some obscure clocking mode"
          # "fetch timestamp from sync unit\nassuming it can be done since we are\nin multiplex mode with no emulation"
          n120 = Unbundle By Name(w139) -> ("awg unit"=w140:T7)
          n121 = Unbundle By Name(w134) -> ("timestamp [s]"=w136:dbl[])
          n122 = call "AWG Get Timestamp.vi"("error in (no error)"=w142, "awg session in"=w140) -> ("error out"=w141:errorcluster, "timestamp [s]"=w135:dbl, "awg session out"=w138:T7)  [unwired: 7 in]
          n123 = Add(x=w135, y=w136) -> (x+y=w133:dbl[])
          n124 = Bundle By Name(cluster=w134, "timestamp [s]"=w133) -> (w132:T1)
          n125 = Bundle By Name(cluster=w139, "awg unit"=w138) -> (w137:T3)
        }
      }
    }
  }
  "error out" <- w35
  "session out" <- w34
  "fetching done?" <- w32
  "aux data" <- w31
  "data packet" <- w30
